vi "SMO.UI.DVRtoRef.vi"(10 "Ref":T1) -> (2 "Ref":u64 format="%016x")   [LabVIEW 2021, in "smo.lvlib" / "SMO.UI.lvclass"]
uses:
  SMO.UI.lvclass
  Typedefs/PrivateData--Ref.ctl
  Typedefs/PrivateData--Cluster.ctl
  Typedefs/PublicEvents--Cluster.ctl
  Typedefs/SMO.UI State--enum.ctl
  Typedefs/PrivateEvents--Cluster.ctl
  SMO.UI.lvclass/SMO.UI.ctl
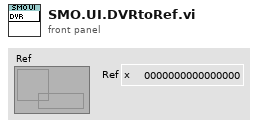
[diagram p1: front panel]
types:
  T1 = typedef "smo.lvlib/SMO.UI.lvclass/PrivateData--Ref.ctl" = refnum<data-value>
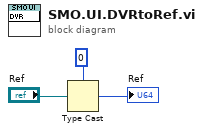
[diagram p0: block diagram]
diagram:
  n1 = Type Cast(type=u64 0 ("Ref"), x="Ref") -> (*(type *) &x=→"Ref":u64)
